vi "NOTHING.vi"(4 "Kinect Depth Data":refnum<queue>, 5 "Event Data":cluster{"sender":refnum<k24>, "e":refnum<k24>}, 6 "Control Ref":refnum<k24>, 7 "Event Common Data":T1) -> ()   [LabVIEW 2011]
uses:
  Microsoft.Kinect
panel:
  in  "User Parameter":variant
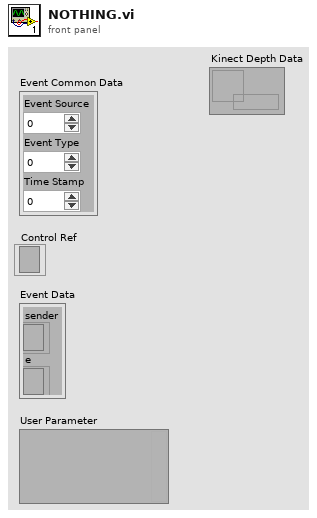
[diagram p1: front panel]
types:
  T1 = cluster{"Event Source":i32, "Event Type":u32, "Time Stamp":u32}
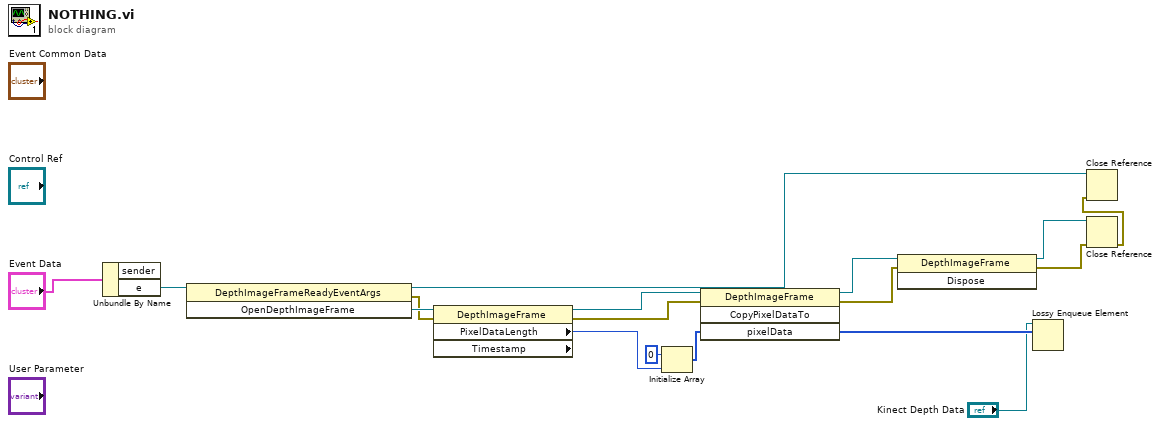
[diagram p0: block diagram]
diagram:
  n1 = Unbundle By Name("Event Data") -> ("e"=w14:refnum<k24>)  [unwired: 1 out]
  n2 = invoke class="DepthImageFrameReadyEventArgs" method="OpenDepthImageFrame"(reference=w14) -> (reference out=w12:refnum<k24>, error out=w15:errorcluster, "OpenDepthImageFrame"=w16:refnum<k24>)  [unwired: 2 in]
  n3 = property on="Property Node" class="DepthImageFrame" props=["PixelDataLength", "Timestamp"](reference=w16, error in=w15) -> (reference out=w7:refnum<k24>, error out=w9:errorcluster, "PixelDataLength"=w1:i32)  [unwired: 1 out]
  n4 = Initialize Array(i16 0 ("element"), w1) -> (w3:i16[])
  n5 = invoke class="DepthImageFrame" method="CopyPixelDataTo"(reference=w7, error in=w9, "pixelData"=w3) -> (reference out=w6:refnum<k24>, error out=w8:errorcluster, "pixelData"=w5:i16[])  [unwired: 1 in, 1 out]
  n6 = invoke class="DepthImageFrame" method="Dispose"(reference=w6, error in=w8) -> (reference out=w13:refnum<k24>, error out=w11:errorcluster)  [unwired: 1 in, 1 out]
  n7 = Lossy Enqueue Element(queue="Kinect Depth Data", element=w5) -> ()  [unwired: 1 in, 4 out]
  n8 = Close Reference(reference=w13, error in (no error)=w11) -> (error out=w10:errorcluster)
  n9 = Close Reference(reference=w12, error in (no error)=w10) -> ()  [unwired: 1 out]
